vi "InitDataSourceVariant.vi"(11 "data source items":T1[](array[typedef])) -> (3 "variant":variant)   [LabVIEW 2017, in "ModbusMaster.lvlib"]
uses:
  <vilib>/addons/InsightCM/Devices/Shared/Common/ModbusMaster/ModbusMaster.lvlib
  <vilib>/addons/InsightCM/MessageBus/Base/controls/DataSourceItem.ctl
  <vilib>/addons/InsightCM/MessageBus/Base/controls/KeyValuePair.ctl
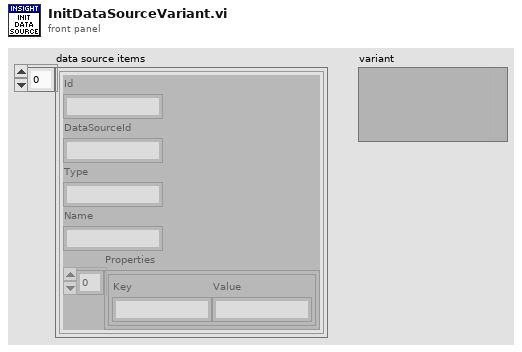
[diagram p1: front panel]
types:
  T1 = typedef "DataSourceItem.ctl" = cluster{"Id":string, "DataSourceId":string, "Type":string, "Name":string, "Properties":T2[]}
  T2 = typedef "KeyValuePair.ctl" = cluster{"Key":string, "Value":string}
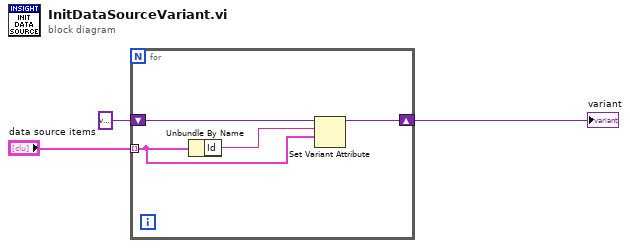
[diagram p0: block diagram]
diagram:
  n1 = for {
    tunnel: "data source items" -> [w4] mode=indexing
    shift-right: [w6] -> w3
    shift-left: variant ("variant") -> [w7]
    n2 = Unbundle By Name(w4) -> ("Id"=w5:string)
    n3 = Set Variant Attribute(Variant=w7, name=w5, value=w4) -> (Variant out=w6:variant)  [unwired: 1 in, 2 out]
  }
  "variant" <- w3
